vi "ConditionalErrorProbe.vi"(1 "error in (no error)":errorcluster) -> (0 "Stop?":bool)   [LabVIEW 2017]
doc: "Displays the error status, code, and description. Allows conditional breakpoints to pause on an error, a warning, or on a particular error code."
panel:
  in  "Tab Control":enum32{"Error   ", "Condition      "}(tab)
  out "Code":i32 format="%#.0f"
  out "Status":bool
  out "Explanation":string
  in  "Cond Code#":i32
  in  "Code 2":bool
  in  "Warning":bool
  in  "Error":bool
  # "Pause if any of the following:"
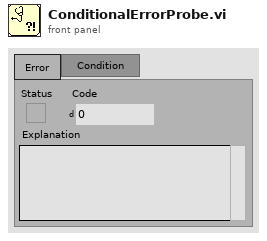
[diagram p1: front panel]
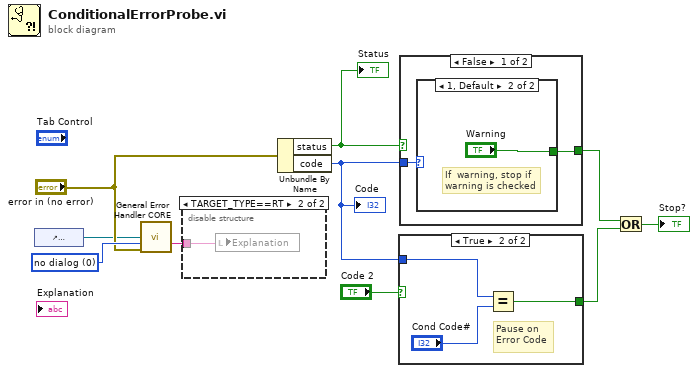
[diagram p0: block diagram]
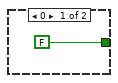
[diagram p3: hidden frame]
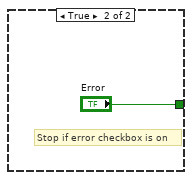
[diagram p4: hidden frame]
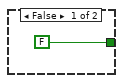
[diagram p5: hidden frame]
diagram:
  w10 = u16 0 items=["no dialog", "OK message", "continue or stop message", "auto error handling dialog", "OK message + warnings", "continue/stop + warnings"] ("type of dialog (OK msg:1)")
  n1 = control-ref of="Explanation"() -> (w8:refnum<vi>)
  n2 = call <vilib>:"General Error Handler CORE.vi"("String to Format (not a refnum)"=w8, "type of dialog (OK msg:1)"=w10, "error in (no error)"="error in (no error)") -> ("message"=w1:string)  [unwired: 7 in, 5 out]
  n3 = disable-structure shown="TARGET_TYPE==RT" {
    disable-tunnel: w1 -> [_ w11]
    frame condition #0 (active) {
    }
    frame condition #1 {
      n4 = local write "Explanation"(w11) -> ()
    }
  }
  n5 = Unbundle By Name("error in (no error)") -> ("status"=w7:bool, "code"=w2:i32)
  "Status" <- w7
  "Code" <- w2
  n6 = case shown="True" "Code 2" {
    tunnel: w2 -> [_ w15]
    tunnel: [FALSE w13] -> w3
    frame False {
    }
    frame True {
      # "Pause on \nError Code"
      n7 = Equal?(x=w15, y="Cond Code#") -> (x = y?=w13:bool)
    }
  }
  n8 = case shown="False" w7 {
    tunnel: [w17 "Error"] -> w6
    tunnel: w2 -> [w16 _]
    frame False {
      n9 = case shown="1, Default" w16 {
        tunnel: [FALSE ("Warning") "Warning"] -> w17
        frame 0 {
        }
        frame 1, Default {
          # "If  warning, stop if warning is checked"
        }
      }
    }
    frame True {
      # "Stop if error checkbox is on"
    }
  }
  n10 = Or(x=w6, y=w3) -> (x .or. y?=→"Stop?":bool)
